vi "DB Create Schema.vi"(8 "error in (no error)":errorcluster, 10 "SQL query":string, 11 "SQLite Database in":refnum<class "SQLite Database.lvclass">) -> (0 "error out":errorcluster, 3 "SQLite Database out":refnum<class "SQLite Database.lvclass">)   [LabVIEW 2023, in "HardwareAbstractionLayer_LVOOP.lvlib" / "SQLite Database.lvclass"]
uses:
  SQLite Database.lvclass
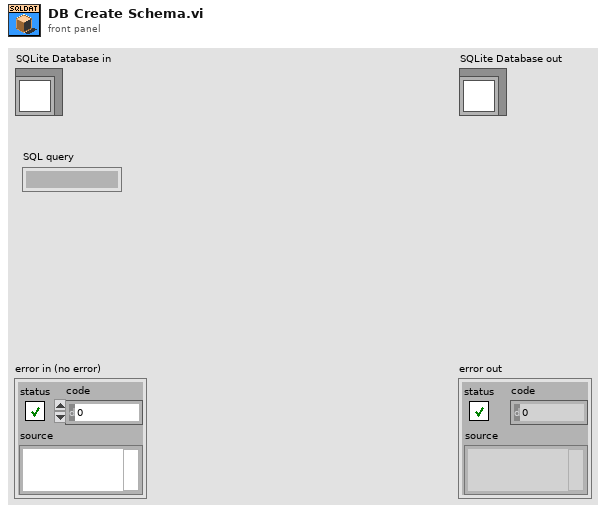
[diagram p1: front panel]
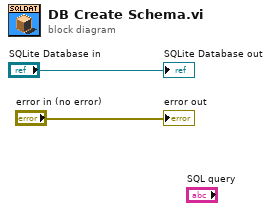
[diagram p0: block diagram]
diagram:
  "error out" <- "error in (no error)"
  "SQLite Database out" <- "SQLite Database in"
